vi "Open Control from Path.vi"(8 "error in (no error)":errorcluster, 11 "ctl path":path) -> (0 "error out":errorcluster, 3 "Value":variant)   [LabVIEW 2019, in "JSON-Schema.lvlib"]
uses:
  JSON-Schema.lvlib
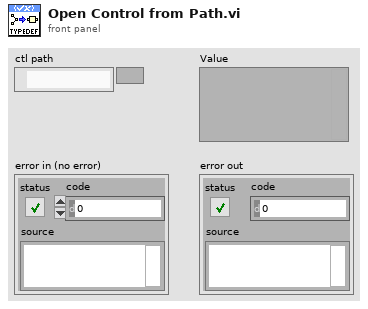
[diagram p1: front panel]
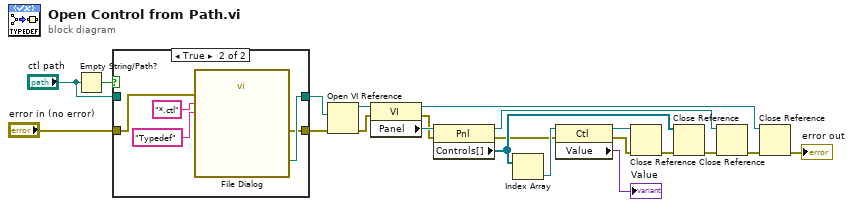
[diagram p0: block diagram]
diagram:
  n1 = Empty String/Path?(string/path="ctl path") -> (empty?=w2:bool)
  n2 = case shown="True" w2 {
    tunnel: [w23 w27] -> w5
    tunnel: "error in (no error)" -> [w22 w26]
    tunnel: [w22 w25] -> w3
    tunnel: "ctl path" -> [w23 _]
    frame False {
    }
    frame True {
      n3 = call "File Dialog"("error in"=w26, "pattern (all files)"="*.ctl", "pattern label"="Typedef") -> ("selected path"=w27:path, "error out"=w25:errorcluster)  [unwired: 9 in, 2 out]
    }
  }
  n4 = Open VI Reference(vi path=w5, error in (no error)=w3) -> (vi reference=w19:refnum<vi>, error out=w14:errorcluster)  [unwired: 4 in]
  n5 = property class="VI"(reference=w19, error in=w14) -> (reference out=w18:refnum<vi>, error out=w9:errorcluster, "Panel"=w21:refnum<vi>)
  n6 = property class="Pnl"(reference=w21, error in=w9) -> (reference out=w16:refnum<vi>, error out=w7:errorcluster, "Controls[]"=w17:refnum<vi>[])
  n7 = Index Array(array=w17) -> (element=w15:refnum<vi>)  [unwired: 1 in]
  n8 = property class="Ctl"(reference=w15, error in=w7) -> (reference out=w11:refnum<vi>, error out=w8:errorcluster, "Value"=→"Value":variant)
  n9 = Close Reference(reference=w11, error in (no error)=w8) -> (error out=w10:errorcluster)
  n10 = Close Reference(reference=w17, error in (no error)=w10) -> (error out=w13:errorcluster)
  n11 = Close Reference(reference=w16, error in (no error)=w13) -> (error out=w12:errorcluster)
  n12 = Close Reference(reference=w18, error in (no error)=w12) -> (error out=→"error out":errorcluster)
